vi "Inject Traverse Pos 2 Inst Pos.vi"() -> (0 "error out":errorcluster, 4 "Path":path)   [LabVIEW 2020]
panel:
  out "Array":path[](array[path])
  out "File Changed":bool
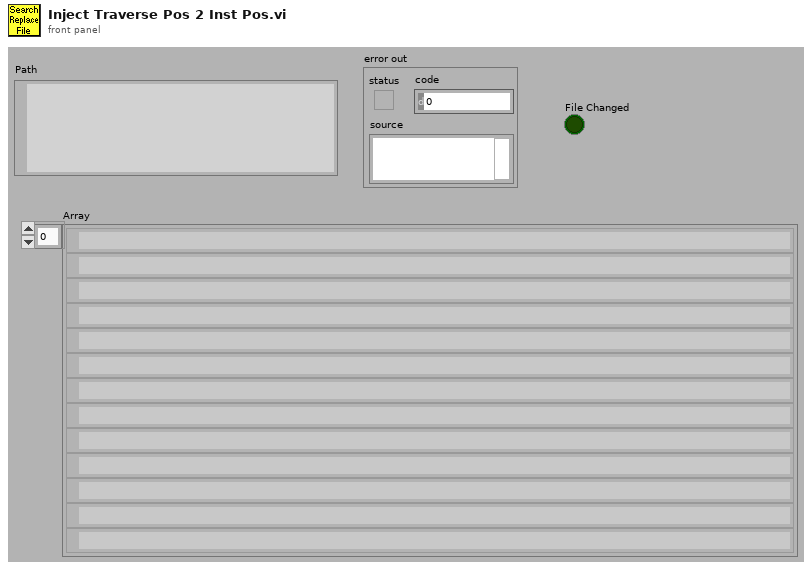
[diagram p1: front panel]
types:
  T1 = enum16{"To Traverse Coordinates", "To User Coordinates"}
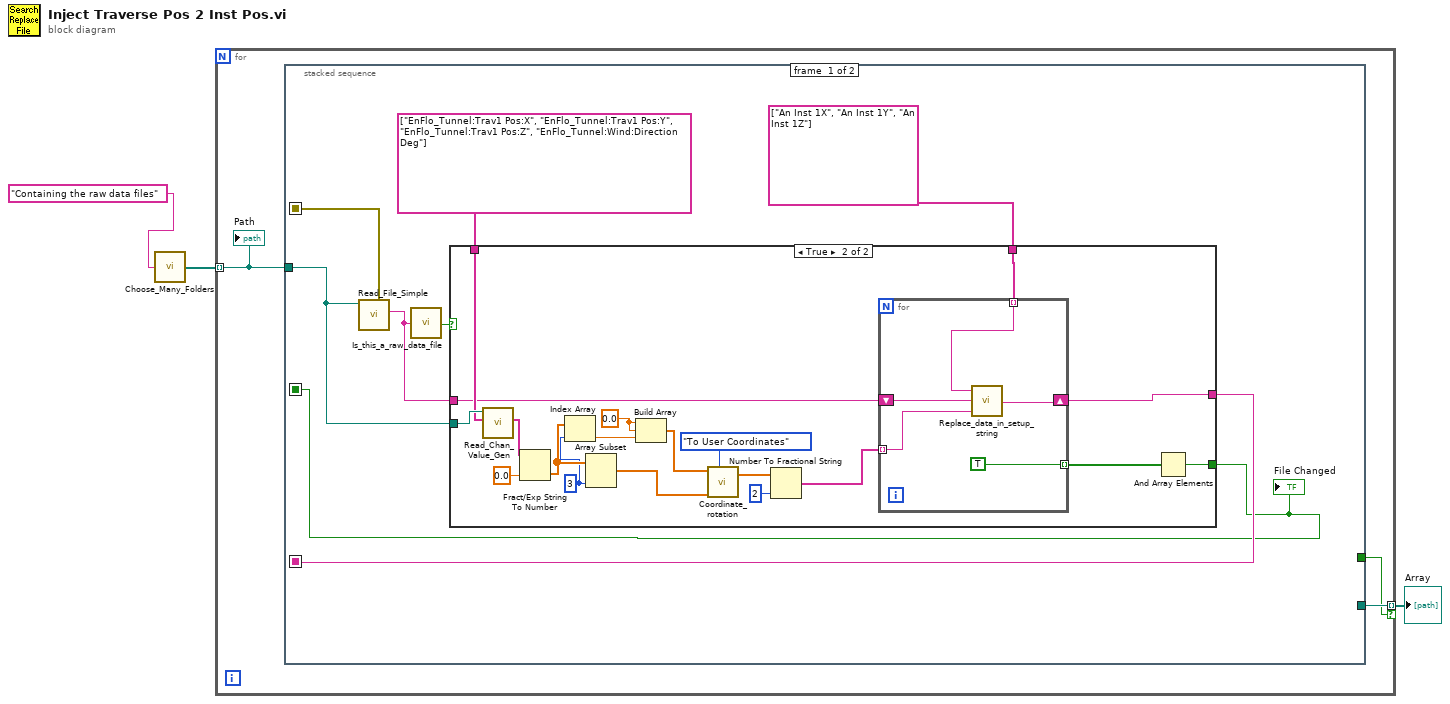
[diagram p0: block diagram]
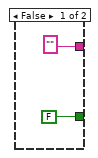
[diagram p2: hidden frame]
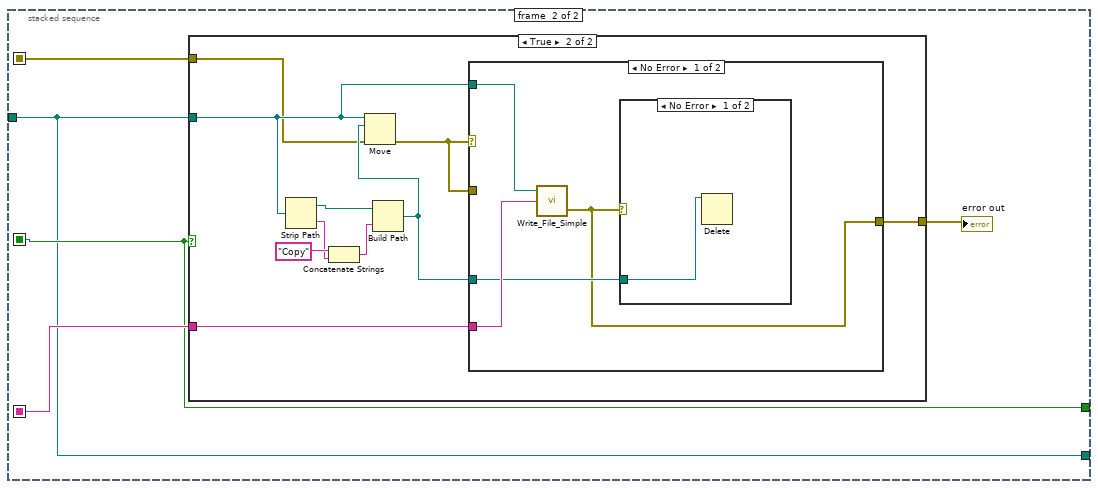
[diagram p3: hidden frame]
diagram:
  n1 = call "Choose_Many_Folders.vi"("Purpose of choosing folder"="Containing the raw data files") -> ("Files"=w2:path[])
  n2 = for {
    tunnel: w2 -> [w6] mode=indexing
    tunnel: [w5] -> w1 mode=indexing if=w4
    n3 = stacked-sequence {
      seq-local: [w14 _] -> [_ w44]
      seq-local: [w12 _] -> [_ w43]
      seq-local: [w11 _] -> [_ w42]
      tunnel: w6 -> [w10 w41]
      tunnel: [_ w41] -> w5
      tunnel: [_ w42] -> w4
      frame #0 {
        n4 = call "Read_File_Simple.vi"("Filename"=w10) -> ("error out"=w14:errorcluster, "string"=w8:string)  [unwired: 4 in, 4 out]
        n5 = call "Is_this_a_raw_data_file.vi"("character string"=w8) -> ("Raw Dat File?"=w7:bool)  [unwired: 2 out]
        n6 = case shown="True" w7 {
          tunnel: string[] ["An Inst 1X", "An Inst 1Y", "An Inst 1Z"] -> [_ w35]
          tunnel: ["" ("string") w34] -> w12
          tunnel: [FALSE w33] -> w11
          tunnel: w10 -> [_ w32]
          tunnel: string[] ["EnFlo_Tunnel:Trav1 Pos:X", "EnFlo_Tunnel:Trav1 Pos:Y", "EnFlo_Tunnel:Trav1 Pos:Z", "EnFlo_Tunnel:Wind:Direction Deg"] -> [_ w31]
          tunnel: w8 -> [_ w30]
          frame False {
          }
          frame True {
            w25 = sgl 0.0 ("default (0 DBL)")
            w23 = 3 ("length")
            n7 = call "Read_Chan_Value_Gen.vi"("Desired Ch Names"=w31, "Raw data file"=w32) -> ("Values"=w28:string[])  [unwired: 9 in]
            n8 = Fract/Exp String To Number(string=w28, default (0 dbl)=sgl 0.0 ("default (0 DBL)")) -> (number=w24:sgl[])  [unwired: 2 in, 1 out]
            n9 = Index Array(array=w24, index=w23) -> (element=w22:sgl)
            n10 = Array Subset(array=w24, length=w23) -> (w27:sgl[])  [unwired: 1 in]
            n11 = Build Array(w25, w25, w22) -> (w21:sgl[])
            n12 = call "Coordinate_rotation.vi"("Roll-Pitch-Yaw"=w21, "Input Position"=w27, "Mode"=T1."To User Coordinates") -> ("Output Position"=w20:sgl[])  [unwired: 2 in, 1 out]
            n13 = Number To Fractional String(number=w20, precision (6)=i16 2) -> (F-format string=w18:string[])  [unwired: 2 in]
            n14 = for {
              shift-right: [w36] -> w34
              shift-left: w30 -> [w39]
              tunnel: w35 -> [w40] mode=indexing
              tunnel: [TRUE] -> w17 mode=indexing
              tunnel: w18 -> [w37] mode=indexing
              n15 = call "Replace_data_in_setup_string.vi"("New data string"=w37, "Input string"=w39, "Variable name"=w40) -> ("Appended string"=w36:string)
            }
            n16 = And Array Elements(Boolean array=w17) -> (logical AND=w33:bool)
          }
        }
        "File Changed" <- w11
      }
      frame #1 {
        n17 = case shown="True" w42 {
          tunnel: w41 -> [_ w52]
          tunnel: w43 -> [_ w51]
          tunnel: [w46 w49] -> w45
          tunnel: w44 -> [w46 w47]
          frame False {
          }
          frame True {
            n18 = Strip Path(path=w52) -> (stripped path=w53:path, name=w55:string)
            n19 = Concatenate Strings("Copy" ("name or relative path"), w55) -> (w54:string)
            n20 = Build Path(base path=w53, name or relative path=w54) -> (appended path=w50:path)
            n21 = Move(source path=w52, error in=w47, 10:w50) -> (error out=w48:errorcluster)  [unwired: 2 in, 2 out]
            n22 = case shown="No Error" w48 {
              tunnel: w52 -> [w60 _]
              tunnel: w51 -> [w59 _]
              tunnel: w50 -> [w58 _]
              tunnel: [w57 w62] -> w49
              tunnel: w48 -> [_ w62]
              frame No Error {
                n23 = call "Write_File_Simple.vi"("character string"=w59, "file path"=w60) -> ("error out"=w57:errorcluster)  [unwired: 1 in, 1 out]
                n24 = case shown="No Error" w57 {
                  tunnel: w58 -> [w61 _]
                  frame No Error {
                    n25 = Delete(path (use dialog)=w61) -> ()  [unwired: 4 in, 3 out]
                  }
                  frame Error {
                  }
                }
              }
              frame Error {
              }
            }
          }
        }
        "error out" <- w45
      }
    }
    "Path" <- w6
  }
  "Array" <- w1
